vi "Begin.vi"(11 "Image Size":T1=enum."320x240") -> (0 "error out":errorcluster)   [LabVIEW 2012]
doc: "Called before other user functions, this VI is expected to open initial I/O refnums, load in file data, and do all program initialization. Notice that the <B>error out</B> terminal is simply used for data flow. Wiring it to other structures or subVIs ensures that this VI runs first."
uses:
  <vilib>/Rock Robotics/WPI/Camera/WPI_CameraImageSize.ctl
  <vilib>/Rock Robotics/WPI/Joystick/WPI_JoystickDeviceEnum.ctl
  <vilib>/Rock Robotics/SystemInterfaces/AI/FPGA_AIGyroChannel.ctl
  Driver/ADXL345 I2C Range.ctl
  <vilib>/Rock Robotics/SystemInterfaces/DIO/FPGA_DIOChannel.ctl
  <vilib>/Rock Robotics/WPI/Encoder/WPI_EncoderType.ctl
  <vilib>/Rock Robotics/SystemInterfaces/DIO/FPGA_DIOPWMChannel.ctl
  <vilib>/Rock Robotics/SystemInterfaces/Typedef/FPGA_TypedefAnalogModuleForGyro.ctl
  <vilib>/Rock Robotics/SystemInterfaces/AI/FPGA_AIChannel.ctl
  <vilib>/Rock Robotics/WPI/Camera/WPI_CameraWhite Balance Values.ctl
  <vilib>/Rock Robotics/WPI/Camera/WPI_CameraExposure Values.ctl
  <vilib>/Rock Robotics/WPI/Camera/WPI_CameraFrameRate.ctl
  <vilib>/Rock Robotics/SystemInterfaces/Typedef/FPGA_TypedefDigitalModule.ctl
  <vilib>/Rock Robotics/WPI/Solenoid/WPI_SolenoidChannel.ctl
  <vilib>/Rock Robotics/SystemInterfaces/Typedef/FPGA_TypedefSolenoidModule.ctl
  <vilib>/Rock Robotics/WPI/Counter/WPI_CounterDigitalInputToDigitalSource.vi
  <vilib>/Rock Robotics/WPI/MotorControl/WPI_MotorControlOpen Jaguar.vi
  <vilib>/Rock Robotics/WPI/MotorControl/WPI_MotorControlOpen Victor.vi
  <vilib>/Rock Robotics/WPI/Counter/WPI_CounterOpen Semi Period Mode.vi
  <vilib>/Rock Robotics/WPI/Solenoid/WPI_SolenoidOpenSingle.vi
  Robot Global Data.vi
panel:
  in  "Encoder Codes\n Per Foot":u16=114
  # "This gets reset in Disable.vi"
  # "114 2011 Robot"
  # "Shooter"
  # "SPEED LOOP DRIVE"
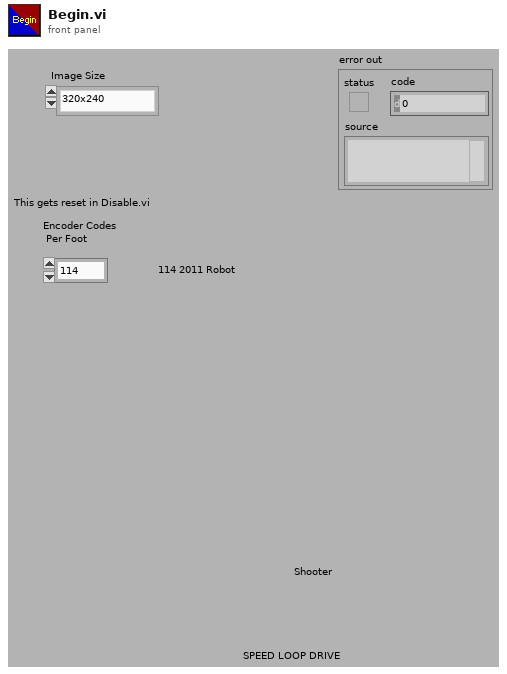
[diagram p1: front panel]
types:
  T1 = typedef "WPI_CameraImageSize.ctl" = enum16{"640x480", "320x240", "160x120"}
  T2 = typedef "FPGA_DIOPWMChannel.ctl" = enum8{"PWM 1", "PWM 2", "PWM 3", "PWM 4", "PWM 5", "PWM 6", "PWM 7", "PWM 8", "PWM 9", "PWM 10", "Invalid"}
  T3 = typedef "FPGA_TypedefDigitalModule.ctl" = enum16{"Digital Module 1", "Digital Module 2"}
  T4 = typedef "FPGA_DIOChannel.ctl" = enum8{"DIO 1", "DIO 2", "DIO 3", "DIO 4", "DIO 5", "DIO 6", "DIO 7", "DIO 8", "DIO 9", "DIO 10", "DIO 11", "DIO 12", "DIO 13", "DIO 14", "Invalid"}
  T5 = typedef "FPGA_TypedefSolenoidModule.ctl" = enum16{"Solenoid Module 1", "Solenoid Module 2"}
  T6 = typedef "WPI_SolenoidChannel.ctl" = enum8{"Solenoid 1", "Solenoid 2", "Solenoid 3", "Solenoid 4", "Solenoid 5", "Solenoid 6", "Solenoid 7", "Solenoid 8", "Invalid"}
  T7 = typedef "WPI_CameraFrameRate.ctl" = u32
  T8 = typedef "WPI_CameraExposure Values.ctl" = enum16{"Auto", "Flicker-free 50 Hz", "Flicker-free 60 Hz", "Hold current"}
  T9 = typedef "WPI_CameraWhite Balance Values.ctl" = enum16{"Auto", "Fixed indoor", "Fixed outdoor 1", "Fixed outdoor 2", "Fixed fluorescent 1", "Fixed fluorescent 2", "Hold current"}
  T10 = typedef "FPGA_AIChannel.ctl" = enum8{"AI 1", "AI 2", "AI 3", "AI 4", "AI 5", "AI 6", "AI 7", "AI 8", "Invalid"}
  T11 = typedef "FPGA_TypedefAnalogModuleForGyro.ctl" = enum16{"Analog Module 1"}
  T12 = typedef "WPI_JoystickDeviceEnum.ctl" = enum16{"USB 1", "USB 2", "USB 3", "USB 4", "Kinect 1", "Kinect 2"}
  T13 = typedef "WPI_EncoderType.ctl" = enum16{"1x", "2x", "4x"}
  T14 = typedef "ADXL345 I2C Range.ctl" = u8
  T15 = typedef "FPGA_AIGyroChannel.ctl" = enum8{"AI 1", "AI 2", "Invalid"}
  T16 = typedef "WPI_DigitalInputDevRef.ctl" = cluster{"DevStatus":errorcluster, "DIO Channel":T4, "Digital Module":T3}
  T17 = typedef "WPI_SolenoidDevRef.ctl" = cluster{"DevStatus":errorcluster, "Solenoid Module":T5, "Forward Solenoid Channel":T6, "Reverse Solenoid Channel":T6}
  T18 = typedef "FPGA_CounterEncoderSourceConvertionLVSourceType.ctl" = cluster{"DevStatus":errorcluster, "AnalogTriggerMode?":bool, "DigitalMode":cluster{"Digital Module":T3, "DIO Channel":T19}, "AnalogTriggerMode":cluster{"AnalogTriggerIndex":T20, "OutputType":T21}}
  T19 = typedef "FPGA_DIODigitalSourceChannel.ctl" = enum8{"DIO 1", "DIO 2", "DIO 3", "DIO 4", "DIO 5", "DIO 6", "DIO 7", "DIO 8", "DIO 9", "DIO 10", "DIO 11", "DIO 12", "DIO 13", "DIO 14", "Disabled"}
  T20 = typedef "FPGA_AnalogTriggerIndex.ctl" = enum8{"Trig 0", "Trig 1", "Trig 2", "Trig 3", "Trig 4", "Trig 5", "Trig 6", "Trig 7", "Invalid"}
  T21 = typedef "FPGA_AnalogTriggerOutType.ctl" = enum16{"InWindow", "TriggerState", "Rising", "Falling"}
  T22 = typedef "WPI_CameraDevRef.ctl" = cluster{"Camera Address":string, "CameraStatus":errorcluster, "Acquire Image Notifier":refnum<notifier>}
  T23 = typedef "WPI_MotorControlDeviceRef.ctl" = cluster{"DeviceStatus":errorcluster, "Type":enum16{"PWM", "CAN"}, "PWM":cluster{"Digital Module":T3, "PWM Channel":T2, "DeadBand":T24}, "CAN":cluster{"Device Number":u8, "Control Mode":T25, "Semaphore":T26, "Max Vout":dbl}, "Invert":bool, "TransformRef":T27, "InvTransformRef":T27}
  T24 = typedef "WPI_PWMDeadband.ctl" = cluster{"Name":string, "maxPositivePwm":i32, "minPositivePwm":i32, "centerPwm":i32, "maxNegativePwm":i32, "minNegativePwm":i32, "angularRange":u16}
  T25 = typedef "WPI_CANJaguar_ControlMode.ctl" = enum8{"Percent VBus", "Current", "Speed", "Position", "Voltage"}
  T26 = typedef "Semaphore RefNum" = refnum<k1>
  T27 = typedef "WPI_PWMTransform_ConPane.ctl" = refnum<vi>
  T28 = typedef "WPI_JoystickDevRef.ctl" = cluster{"Device":T12}
  T29 = typedef "WPI_CounterDevRef.ctl" = cluster{"DevStatus":errorcluster, "CntIndex":T30}
  T30 = typedef "FPGA_CounterCtrSystemIndex.ctl" = enum8{"Ctr 0", "Ctr 1", "Ctr 2", "Ctr 3", "Ctr 4", "Ctr 5", "Ctr 6", "Ctr 7", "Invalid"}
  T31 = typedef "WPI_I2CDevRef.ctl" = cluster{"DevStatus":errorcluster, "Digital Module":T3, "Device Address":u8}
  T32 = typedef "WPI_GyroDevRef.ctl" = cluster{"DevStatus":errorcluster, "Analog Module":T33, "Analog Channel":T10, "Offset":dbl, "Gain (VoltsPerDegree/Second)":dbl}
  T33 = typedef "FPGA_TypedefAnalogModule.ctl" = enum16{"Analog Module 1", "Analog Module 2"}
  T34 = typedef "WPI_AnalogChannelDevRef.ctl" = cluster{"DevStatus":errorcluster, "Analog Module":T33, "Analog Channel":T10}
  T35 = typedef "WPI_EncoderDevRef.ctl" = cluster{"DevStatus":errorcluster, "EncoderIndex":T36, "CounterIndex":T30, "DistancePerCount":dbl, "Decoding Type":T13}
  T36 = typedef "FPGA_EncoderIdx.ctl" = enum8{"Enc 0", "Enc 1", "Enc 2", "Enc 3", "Invalid"}
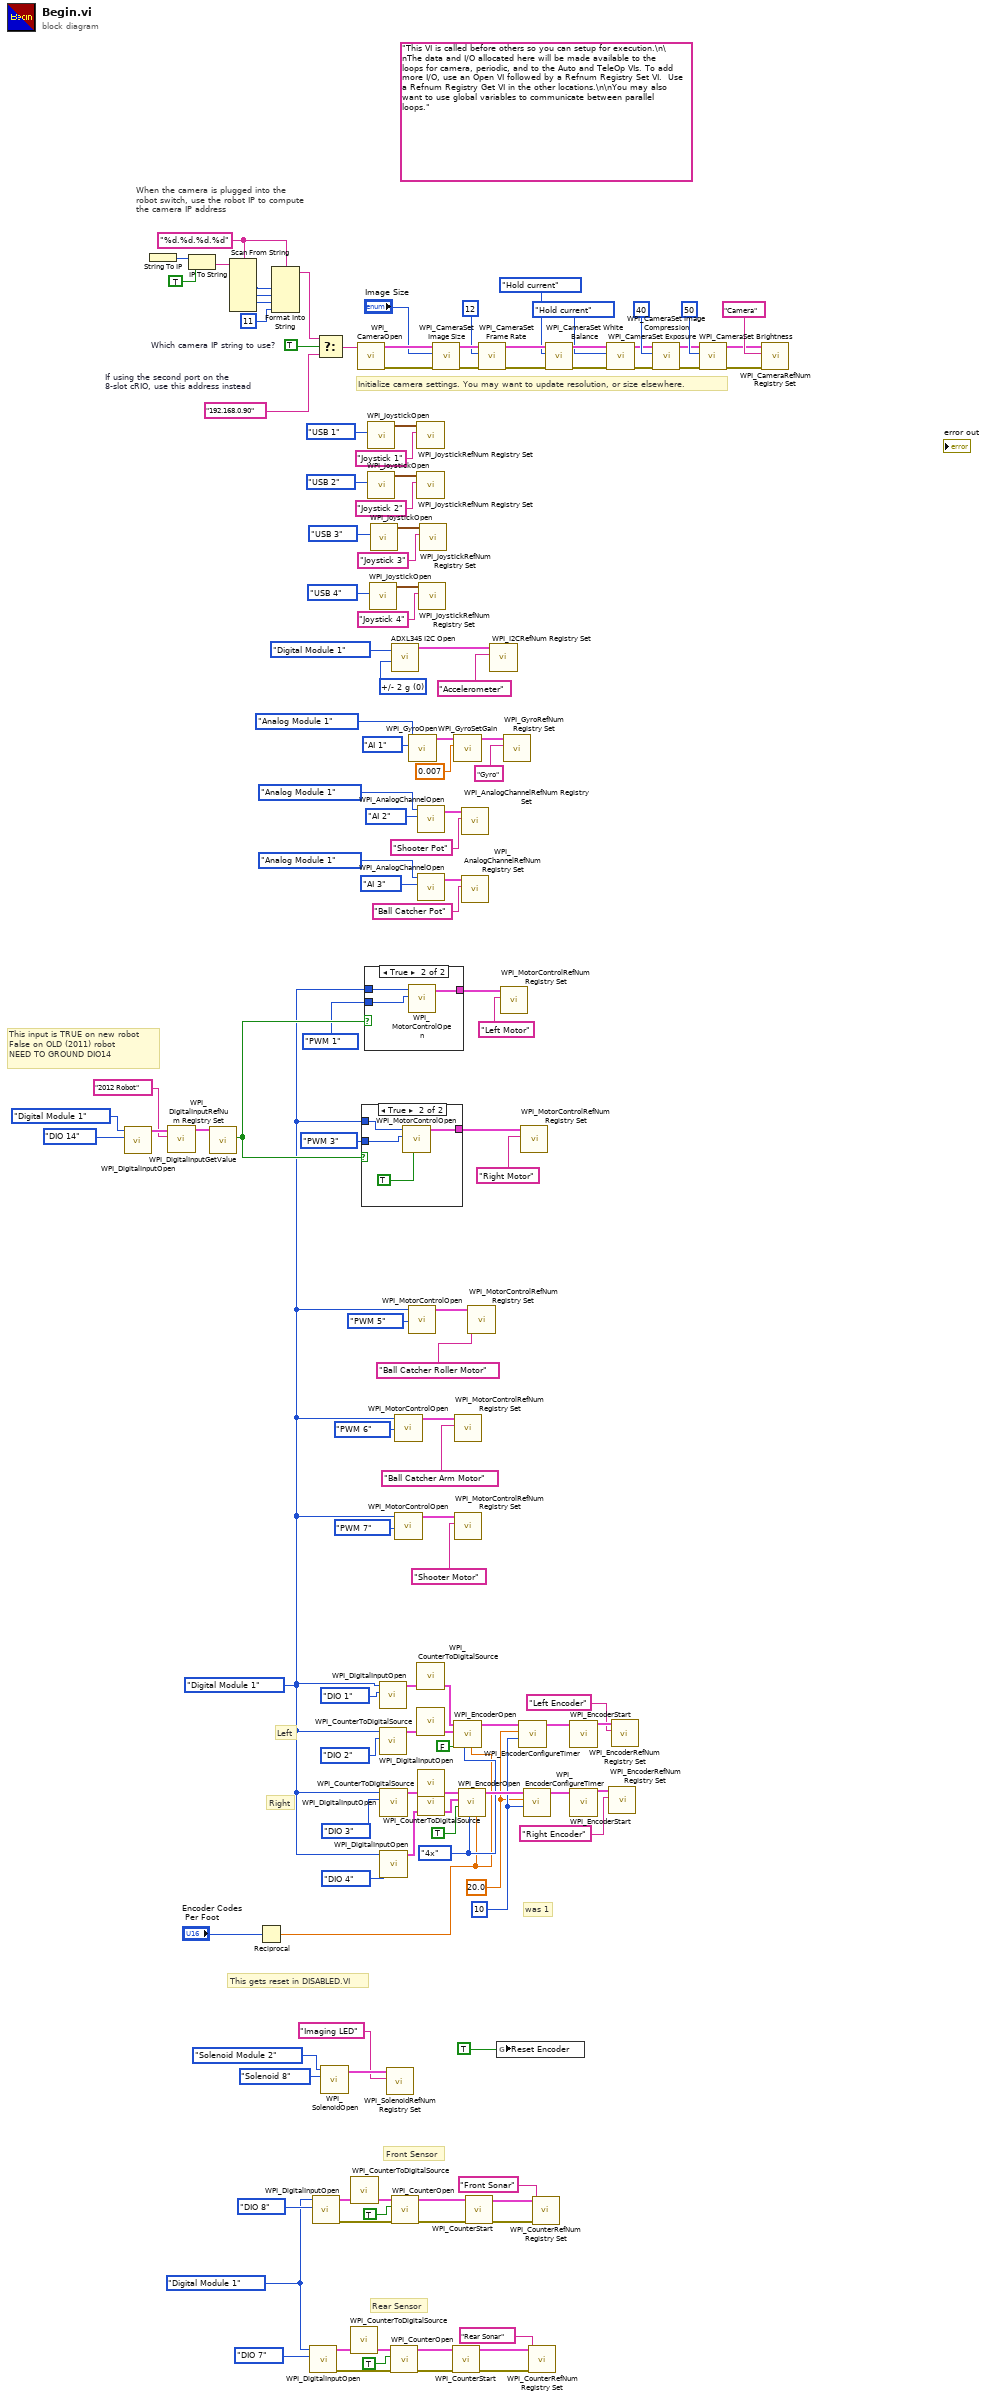
[diagram p0: block diagram]
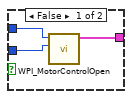
[diagram p2: hidden frame]
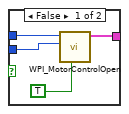
[diagram p3: hidden frame]
diagram:
  w19 = FPGA_TypedefDigitalModule."Digital Module 1" ("DIO Module")
  w40 = TRUE  # Which camera IP string to use?
  w44 = "%d.%d.%d.%d" ("format string")
  w41 = "192.168.0.90"  # If using the second port on the 8-slot cRIO, use this address instead
  (unwired) "This VI is called before others so you can setup for execution.\n\nThe data and I/O allocated here will be made available to the loops for camera, periodic, and to the Auto and TeleOp VIs. To add more I/O, use an Open VI followed by a Refnum Registry Set VI.  Use a Refnum Registry Get VI in the other locations.\n\nYou may also want to use global variables to communicate between parallel loops."
  w110 = u8 10 ("Number Samples to Average")
  w109 = 20.0 ("Minimum Rate")
  w103 = WPI_EncoderType."4x" ("Decoding Type")
  w2 = FPGA_TypedefDigitalModule."Digital Module 1" ("DIO Module")
  w128 = T14 0 items=["+/- 2 g", "+/- 4 g", "+/- 8 g", "+/- 16 g"] ("Range")
  # "This input is TRUE on new robot\nFalse on OLD (2011) robot \nNEED TO GROUND DIO14"
  # "This gets reset in DISABLED.VI"
  # "Rear Sensor"
  # "Front Sensor"
  # "When the camera is plugged into the\nrobot switch, use the robot IP to compute\nthe camera IP address"
  # "Initialize camera settings. You may want to update resolution, or size elsewhere."
  # "was 1"
  # "Right"
  # "Left"
  n1 = call <vilib>:"WPI_DigitalInputOpen.vi"("DIO Channel"=FPGA_DIOChannel."DIO 14", "Digital Module (Module 1)"=FPGA_TypedefDigitalModule."Digital Module 1") -> ("DigitalInputDevRef"=w13:T16)  [unwired: 1 in, 8 out]
  n2 = String To IP() -> (0:w51:u32)  [unwired: 1 in]
  n3 = call <vilib>:"WPI_DigitalInputRefNum Registry Set.vi"("refnum name"="2012 Robot", "DigitalInputDevRef"=w13) -> ("DigitalInputDevRef"=w10:T16)  [unwired: 8 in, 1 out]
  n4 = IP To String(1:TRUE ("dot notation? (F)"), 2:w51) -> (0:w49:string)
  n5 = call <vilib>:"WPI_DigitalInputGetValue.vi"("DigitalInputDevRef"=w10) -> ("Value"=w9:bool)  [unwired: 8 in, 2 out]
  n6 = Scan From String(format string=w44, input string=w49) -> (output 1=w48:i32, output 2=w47:i32, output 3=w46:i32)  [unwired: 7 in, 3 out]
  n7 = Reciprocal(x="Encoder Codes\n Per Foot") -> (1/x=w102:dbl)
  n8 = Format Into String(format string=w44, w48, w47, w46, 11 ("Compression")) -> (resulting string=w42:string)  [unwired: 2 in, 1 out]
  n9 = call <vilib>:"WPI_DigitalInputOpen.vi"("DIO Channel"=FPGA_DIOChannel."DIO 7", "Digital Module (Module 1)"=w19) -> ("error out"=w29:errorcluster, "DigitalInputDevRef"=w27:T16)  [unwired: 1 in, 7 out]
  n10 = call <vilib>:"WPI_DigitalInputOpen.vi"("DIO Channel"=FPGA_DIOChannel."DIO 8", "Digital Module (Module 1)"=w19) -> ("error out"=w31:errorcluster, "DigitalInputDevRef"=w37:T16)  [unwired: 1 in, 7 out]
  n11 = Select(t=w42, s=w40, f=w41) -> (s? t:f=w43:string)
  n12 = call-poly <vilib>:"WPI_SolenoidOpen.vi"("Solenoid Channel"=WPI_SolenoidChannel."Solenoid 8", "Solenoid Module (Module 1)"=FPGA_TypedefSolenoidModule."Solenoid Module 2") -> ("SolenoidDevRef"=w16:T17)  [unwired: 1 in, 8 out]
  n13 = call-poly <vilib>:"WPI_CounterToDigitalSource.vi"("DigitalInputDevRef"=w27) -> ("Digital Source"=w35:T18)  [unwired: 6 in]
  n14 = call-poly <vilib>:"WPI_CounterToDigitalSource.vi"("DigitalInputDevRef"=w37) -> ("Digital Source"=w39:T18)  [unwired: 6 in]
  n15 = call <vilib>:"WPI_CameraOpen.vi"("Camera Address"=w43) -> ("error out"=w63:errorcluster, "CameraDevRef"=w64:T22)  [unwired: 1 in, 8 out]
  n16 = case shown="True" w9 {
    tunnel: [w141 w145] -> w7
    tunnel: FPGA_DIOPWMChannel."PWM 3" ("Motor PWM Channel 2") -> [w140 w143]
    tunnel: w2 -> [w139 w144]
    frame False {
      n17 = call-poly <vilib>:"WPI_MotorControlOpen.vi"("PWM Channel"=w140, "Digital Module (Module 1)"=w139) -> ("MotorControlDeviceRef"=w141:T23)  [unwired: 5 in, 4 out]
    }
    frame True {
      n18 = call-poly <vilib>:"WPI_MotorControlOpen.vi"("Invert"=TRUE, "PWM Channel"=w143, "Digital Module (Module 1)"=w144) -> ("MotorControlDeviceRef"=w145:T23)  [unwired: 4 in, 4 out]
    }
  }
  n19 = case shown="True" w9 {
    tunnel: [w148 w152] -> w5
    tunnel: FPGA_DIOPWMChannel."PWM 1" ("Motor PWM Channel") -> [w147 w151]
    tunnel: w2 -> [w146 w150]
    frame False {
      n20 = call-poly <vilib>:"WPI_MotorControlOpen.vi"("Invert"=TRUE, "PWM Channel"=w147, "Digital Module (Module 1)"=w146) -> ("MotorControlDeviceRef"=w148:T23)  [unwired: 4 in, 4 out]
    }
    frame True {
      n21 = call-poly <vilib>:"WPI_MotorControlOpen.vi"("PWM Channel"=w151, "Digital Module (Module 1)"=w150) -> ("MotorControlDeviceRef"=w152:T23)  [unwired: 5 in, 4 out]
    }
  }
  n22 = call <vilib>:"WPI_JoystickOpen.vi"("JoystickDevice"=WPI_JoystickDeviceEnum."USB 1") -> ("JoystickDevRef"=w138:T28)  [unwired: 10 in]
  n23 = call <vilib>:"WPI_JoystickOpen.vi"("JoystickDevice"=WPI_JoystickDeviceEnum."USB 2") -> ("JoystickDevRef"=w135:T28)  [unwired: 10 in]
  n24 = call <vilib>:"WPI_JoystickOpen.vi"("JoystickDevice"=WPI_JoystickDeviceEnum."USB 4") -> ("JoystickDevRef"=w89:T28)  [unwired: 10 in]
  n25 = call <vilib>:"WPI_JoystickOpen.vi"("JoystickDevice"=WPI_JoystickDeviceEnum."USB 3") -> ("JoystickDevRef"=w92:T28)  [unwired: 10 in]
  n26 = call <vilib>:"WPI_DigitalInputOpen.vi"("DIO Channel"=FPGA_DIOChannel."DIO 1" ("Encoder A Channel"), "Digital Module (Module 1)"=w2) -> ("DigitalInputDevRef"=w94:T16)  [unwired: 1 in, 8 out]
  n27 = call <vilib>:"WPI_DigitalInputOpen.vi"("DIO Channel"=FPGA_DIOChannel."DIO 2" ("Encoder B Channel"), "Digital Module (Module 1)"=w2) -> ("DigitalInputDevRef"=w93:T16)  [unwired: 1 in, 8 out]
  n28 = call <vilib>:"WPI_DigitalInputOpen.vi"("DIO Channel"=FPGA_DIOChannel."DIO 3" ("Encoder A Channel"), "Digital Module (Module 1)"=w2) -> ("DigitalInputDevRef"=w86:T16)  [unwired: 1 in, 8 out]
  n29 = call <vilib>:"WPI_DigitalInputOpen.vi"("DIO Channel"=FPGA_DIOChannel."DIO 4" ("Encoder B Channel"), "Digital Module (Module 1)"=w2) -> ("DigitalInputDevRef"=w85:T16)  [unwired: 1 in, 8 out]
  n30 = call <vilib>:"WPI_SolenoidRefNum Registry Set.vi"("refnum name"="Imaging LED", "SolenoidDevRef"=w16) -> ()  [unwired: 8 in, 2 out]
  n31 = call-poly <vilib>:"WPI_CounterOpen.vi"("error in (no error)"=w29, "High Pulse (T)"=TRUE, "Source"=w35) -> ("error out"=w28:errorcluster, "CounterDevRef"=w34:T29)  [unwired: 7 in]
  n32 = call "ADXL345 I2C Open.vi"("Range"=w128, "DIO Module (Slot 4)"=FPGA_TypedefDigitalModule."Digital Module 1" ("DIO Module")) -> ("I2CDevRef"=w129:T31)  [unwired: 2 in, 7 out]
  n33 = call-poly <vilib>:"WPI_CounterOpen.vi"("error in (no error)"=w31, "High Pulse (T)"=TRUE, "Source"=w39) -> ("error out"=w30:errorcluster, "CounterDevRef"=w38:T29)  [unwired: 7 in]
  n34 = call-poly <vilib>:"WPI_MotorControlOpen.vi"("PWM Channel"=FPGA_DIOPWMChannel."PWM 6" ("Motor PWM Channel 2"), "Digital Module (Module 1)"=w2) -> ("MotorControlDeviceRef"=w80:T23)  [unwired: 5 in, 4 out]
  n35 = call-poly <vilib>:"WPI_MotorControlOpen.vi"("PWM Channel"=FPGA_DIOPWMChannel."PWM 7" ("Motor PWM Channel 2"), "Digital Module (Module 1)"=w2) -> ("MotorControlDeviceRef"=w99:T23)  [unwired: 5 in, 4 out]
  n36 = call-poly <vilib>:"WPI_MotorControlOpen.vi"("PWM Channel"=FPGA_DIOPWMChannel."PWM 5" ("Motor PWM Channel 2"), "Digital Module (Module 1)"=w2) -> ("MotorControlDeviceRef"=w83:T23)  [unwired: 5 in, 4 out]
  n37 = call <vilib>:"WPI_GyroOpen.vi"("Analog Channel"=FPGA_AIGyroChannel."AI 1" ("Channel 2"), "Analog Module (Module 1)"=FPGA_TypedefAnalogModuleForGyro."Analog Module 1" ("Analog Module 2")) -> ("GyroDevRef"=w124:T32)  [unwired: 4 in, 5 out]
  n38 = call <vilib>:"WPI_JoystickRefNum Registry Set.vi"("refnum name"="Joystick 1", "JoystickDevRef"=w138) -> ()  [unwired: 8 in, 2 out]
  n39 = call <vilib>:"WPI_JoystickRefNum Registry Set.vi"("refnum name"="Joystick 2", "JoystickDevRef"=w135) -> ()  [unwired: 8 in, 2 out]
  n40 = call-poly <vilib>:"WPI_CounterToDigitalSource.vi"("DigitalInputDevRef"=w94) -> ("Digital Source"=w121:T18)  [unwired: 6 out]
  n41 = call-poly <vilib>:"WPI_CounterToDigitalSource.vi"("DigitalInputDevRef"=w93) -> ("Digital Source"=w122:T18)  [unwired: 6 out]
  n42 = call <vilib>:"WPI_AnalogChannelOpen.vi"("Analog Channel"=FPGA_AIChannel."AI 2", "Analog Module (Module 1)"=FPGA_TypedefAnalogModuleForGyro."Analog Module 1" ("Analog Module 2")) -> ("AIDeviceRef"=w95:T34)  [unwired: 1 in, 8 out]
  n43 = call <vilib>:"WPI_AnalogChannelOpen.vi"("Analog Channel"=FPGA_AIChannel."AI 3", "Analog Module (Module 1)"=FPGA_TypedefAnalogModuleForGyro."Analog Module 1" ("Analog Module 2")) -> ("AIDeviceRef"=w76:T34)  [unwired: 1 in, 8 out]
  n44 = call-poly <vilib>:"WPI_CounterToDigitalSource.vi"("DigitalInputDevRef"=w86) -> ("Digital Source"=w115:T18)  [unwired: 6 out]
  n45 = call-poly <vilib>:"WPI_CounterToDigitalSource.vi"("DigitalInputDevRef"=w85) -> ("Digital Source"=w116:T18)  [unwired: 6 out]
  n46 = call <vilib>:"WPI_JoystickRefNum Registry Set.vi"("refnum name"="Joystick 4", "JoystickDevRef"=w89) -> ()  [unwired: 8 in, 2 out]
  n47 = call <vilib>:"WPI_JoystickRefNum Registry Set.vi"("refnum name"="Joystick 3", "JoystickDevRef"=w92) -> ()  [unwired: 8 in, 2 out]
  n48 = call <vilib>:"WPI_CameraSet Image Size.vi"("error in (no error)"=w63, "Image Size"="Image Size", "CameraDevRef"=w64) -> ("error out"=w62:errorcluster, "CameraDevRef Out"=w65:T22)  [unwired: 7 out]
  n49 = call <vilib>:"WPI_CounterStart.vi"("error in (no error)"=w28, "CounterDevRef in"=w34) -> ("error out"=w22:errorcluster, "CounterDevRef out"=w23:T29)  [unwired: 8 in]
  n50 = call <vilib>:"WPI_GyroSetGain.vi"("Gain (VoltsPerDegree/Second)"=0.007 ("Gain (VoltsPerDegree/Second) 2"), "GyroDevRef"=w124) -> ("GyroDevRef"=w131:T32)  [unwired: 1 in, 8 out]
  n51 = call <vilib>:"WPI_EncoderOpen.vi"("DistancePerCount"=w102, "Decoding Type"=w103, "Invert Direction (False)"=FALSE, "BSource"=w122, "ASource"=w121) -> ("EncoderDevRef"=w117:T35)  [unwired: 3 in, 3 out]
  n52 = call <vilib>:"WPI_MotorControlRefNum Registry Set.vi"("refnum name"="Ball Catcher Arm Motor", "MotorControlDevRef"=w80) -> ()  [unwired: 8 in, 2 out]
  n53 = call <vilib>:"WPI_MotorControlRefNum Registry Set.vi"("refnum name"="Shooter Motor", "MotorControlDevRef"=w99) -> ()  [unwired: 8 in, 2 out]
  n54 = call <vilib>:"WPI_EncoderOpen.vi"("DistancePerCount"=w102, "Decoding Type"=w103, "Invert Direction (False)"=TRUE, "BSource"=w116, "ASource"=w115) -> ("EncoderDevRef"=w111:T35)  [unwired: 3 in, 3 out]
  n55 = call <vilib>:"WPI_AnalogChannelRefNum Registry Set.vi"("refnum name"="Shooter Pot", "AIDeviceRef"=w95) -> ()  [unwired: 8 in, 2 out]
  n56 = call <vilib>:"WPI_AnalogChannelRefNum Registry Set.vi"("refnum name"="Ball Catcher Pot", "AIDeviceRef"=w76) -> ()  [unwired: 8 in, 2 out]
  n57 = call <vilib>:"WPI_CounterStart.vi"("error in (no error)"=w30, "CounterDevRef in"=w38) -> ("error out"=w24:errorcluster, "CounterDevRef out"=w25:T29)  [unwired: 8 in]
  n58 = call <vilib>:"WPI_MotorControlRefNum Registry Set.vi"("refnum name"="Ball Catcher Roller Motor", "MotorControlDevRef"=w83) -> ()  [unwired: 8 in, 2 out]
  n59 = call <vilib>:"WPI_CameraSet Frame Rate.vi"("error in (no error)"=w62, "Frame Rate (fps)"=T7 12, "CameraDevRef"=w65) -> ("error out"=w61:errorcluster, "CameraDevRef Out"=w67:T22)  [unwired: 7 out]
  n60 = call <vilib>:"WPI_I2CRefNum Registry Set.vi"("refnum name"="Accelerometer", "I2CDevRef"=w129) -> ()  [unwired: 8 in, 2 out]
  n61 = global write "Robot Global Data.vi" "Reset Encoder"(TRUE ("Reset Encoder")) -> ()
  n62 = call <vilib>:"WPI_MotorControlRefNum Registry Set.vi"("refnum name"="Left Motor", "MotorControlDevRef"=w5) -> ()  [unwired: 8 in, 2 out]
  n63 = call <vilib>:"WPI_GyroRefNum Registry Set.vi"("refnum name"="Gyro", "GyroDevRef"=w131) -> ()  [unwired: 8 in, 2 out]
  n64 = call <vilib>:"WPI_EncoderConfigureTimer.vi"("Number Samples to Average"=w110, "Minimum Rate"=w109, "EncoderDevRef"=w117) -> ("EncoderDevRef"=w118:T35)  [unwired: 1 in, 7 out]
  n65 = call <vilib>:"WPI_MotorControlRefNum Registry Set.vi"("refnum name"="Right Motor", "MotorControlDevRef"=w7) -> ()  [unwired: 8 in, 2 out]
  n66 = call <vilib>:"WPI_EncoderConfigureTimer.vi"("Number Samples to Average"=w110, "Minimum Rate"=w109, "EncoderDevRef"=w111) -> ("EncoderDevRef"=w112:T35)  [unwired: 1 in, 7 out]
  n67 = call <vilib>:"WPI_CounterRefNum Registry Set.vi"("error in (no error)"=w22, "refnum name"="Rear Sonar", "CounterDevRef"=w23) -> ()  [unwired: 7 in, 2 out]
  n68 = call <vilib>:"WPI_CounterRefNum Registry Set.vi"("error in (no error)"=w24, "refnum name"="Front Sonar", "CounterDevRef"=w25) -> ()  [unwired: 7 in, 2 out]
  n69 = call <vilib>:"WPI_CameraSet White Balance.vi"("error in (no error)"=w61, "White Balance"=WPI_CameraWhite_Balance_Values."Hold current", "CameraDevRef"=w67) -> ("error out"=w60:errorcluster, "CameraDevRef Out"=w66:T22)  [unwired: 7 out]
  n70 = call <vilib>:"WPI_EncoderStart.vi"("EncoderDevRef"=w118) -> ("EncoderDevRef"=w107:T35)  [unwired: 1 in, 9 out]
  n71 = call <vilib>:"WPI_EncoderStart.vi"("EncoderDevRef"=w112) -> ("EncoderDevRef"=w105:T35)  [unwired: 1 in, 9 out]
  n72 = call <vilib>:"WPI_CameraSet Exposure.vi"("error in (no error)"=w60, "Exposure"=WPI_CameraExposure_Values."Hold current", "CameraDevRef"=w66) -> ("error out"=w59:errorcluster, "CameraDevRef Out"=w69:T22)  [unwired: 7 out]
  n73 = call <vilib>:"WPI_EncoderRefNum Registry Set.vi"("refnum name"="Right Encoder", "EncoderDevRef"=w105) -> ()  [unwired: 8 in, 2 out]
  n74 = call <vilib>:"WPI_EncoderRefNum Registry Set.vi"("refnum name"="Left Encoder", "EncoderDevRef"=w107) -> ()  [unwired: 8 in, 2 out]
  n75 = call <vilib>:"WPI_CameraSet Image Compression.vi"("error in (no error)"=w59, "Compression"=40, "CameraDevRef"=w69) -> ("error out"=w58:errorcluster, "CameraDevRef Out"=w68:T22)  [unwired: 7 out]
  n76 = call <vilib>:"WPI_CameraSet Brightness.vi"("error in (no error)"=w58, "Brightness"=50, "CameraDevRef"=w68) -> ("error out"=w56:errorcluster, "CameraDevRef Out"=w57:T22)  [unwired: 7 out]
  n77 = call <vilib>:"WPI_CameraRefNum Registry Set.vi"("error in (no error)"=w56, "refnum name"="Camera", "CameraDevRef"=w57) -> ()  [unwired: 9 out]
